vi "大富翁.vi"() -> ()   [LabVIEW 2014] (continued)
      n525 = property on="30房1" class="Bool (strict)"("Visible"=w18) -> ()  [unwired: 2 in, 2 out]
      n526 = property on="30房2" class="Bool (strict)"("Visible"=w18) -> ()  [unwired: 2 in, 2 out]
      n527 = property on="30房3" class="Bool (strict)"("Visible"=w18) -> ()  [unwired: 2 in, 2 out]
      n528 = property on="30房4" class="Bool (strict)"("Visible"=w18) -> ()  [unwired: 2 in, 2 out]
      n529 = property on="30旅1" class="Bool (strict)"("Visible"=w18) -> ()  [unwired: 2 in, 2 out]
      n530 = property on="30旅2" class="Bool (strict)"("Visible"=w18) -> ()  [unwired: 2 in, 2 out]
      n531 = property on="30旅3" class="Bool (strict)"("Visible"=w18) -> ()  [unwired: 2 in, 2 out]
      n532 = property on="30旅4" class="Bool (strict)"("Visible"=w18) -> ()  [unwired: 2 in, 2 out]
      n533 = property on="31房1" class="Bool (strict)"("Visible"=w18) -> ()  [unwired: 2 in, 2 out]
      n534 = property on="31房2" class="Bool (strict)"("Visible"=w18) -> ()  [unwired: 2 in, 2 out]
      n535 = property on="31房3" class="Bool (strict)"("Visible"=w18) -> ()  [unwired: 2 in, 2 out]
      n536 = property on="31房4" class="Bool (strict)"("Visible"=w18) -> ()  [unwired: 2 in, 2 out]
      n537 = property on="31旅1" class="Bool (strict)"("Visible"=w18) -> ()  [unwired: 2 in, 2 out]
      n538 = property on="31旅2" class="Bool (strict)"("Visible"=w18) -> ()  [unwired: 2 in, 2 out]
      n539 = property on="31旅3" class="Bool (strict)"("Visible"=w18) -> ()  [unwired: 2 in, 2 out]
      n540 = property on="31旅4" class="Bool (strict)"("Visible"=w18) -> ()  [unwired: 2 in, 2 out]
      n541 = property on="33房1" class="Bool (strict)"("Visible"=w17) -> ()  [unwired: 2 in, 2 out]
      n542 = property on="33房2" class="Bool (strict)"("Visible"=w17) -> ()  [unwired: 2 in, 2 out]
      n543 = property on="33房3" class="Bool (strict)"("Visible"=w17) -> ()  [unwired: 2 in, 2 out]
      n544 = property on="33房4" class="Bool (strict)"("Visible"=w17) -> ()  [unwired: 2 in, 2 out]
      n545 = property on="33旅1" class="Bool (strict)"("Visible"=w17) -> ()  [unwired: 2 in, 2 out]
      n546 = property on="33旅2" class="Bool (strict)"("Visible"=w17) -> ()  [unwired: 2 in, 2 out]
      n547 = property on="33旅3" class="Bool (strict)"("Visible"=w17) -> ()  [unwired: 2 in, 2 out]
      n548 = property on="33旅4" class="Bool (strict)"("Visible"=w17) -> ()  [unwired: 2 in, 2 out]
      n549 = property on="34房1" class="Bool (strict)"("Visible"=w17) -> ()  [unwired: 2 in, 2 out]
      n550 = property on="34房2" class="Bool (strict)"("Visible"=w17) -> ()  [unwired: 2 in, 2 out]
      n551 = property on="34房3" class="Bool (strict)"("Visible"=w17) -> ()  [unwired: 2 in, 2 out]
      n552 = property on="34房4" class="Bool (strict)"("Visible"=w17) -> ()  [unwired: 2 in, 2 out]
      n553 = property on="34旅1" class="Bool (strict)"("Visible"=w17) -> ()  [unwired: 2 in, 2 out]
      n554 = property on="34旅2" class="Bool (strict)"("Visible"=w17) -> ()  [unwired: 2 in, 2 out]
      n555 = property on="34旅3" class="Bool (strict)"("Visible"=w17) -> ()  [unwired: 2 in, 2 out]
      n556 = property on="34旅4" class="Bool (strict)"("Visible"=w17) -> ()  [unwired: 2 in, 2 out]
      n557 = property on="36房1" class="Bool (strict)"("Visible"=w17) -> ()  [unwired: 2 in, 2 out]
      n558 = property on="36房2" class="Bool (strict)"("Visible"=w17) -> ()  [unwired: 2 in, 2 out]
      n559 = property on="36房3" class="Bool (strict)"("Visible"=w17) -> ()  [unwired: 2 in, 2 out]
      n560 = property on="36房4" class="Bool (strict)"("Visible"=w17) -> ()  [unwired: 2 in, 2 out]
      n561 = property on="36旅1" class="Bool (strict)"("Visible"=w17) -> ()  [unwired: 2 in, 2 out]
      n562 = property on="36旅2" class="Bool (strict)"("Visible"=w17) -> ()  [unwired: 2 in, 2 out]
      n563 = property on="36旅3" class="Bool (strict)"("Visible"=w17) -> ()  [unwired: 2 in, 2 out]
      n564 = property on="36旅4" class="Bool (strict)"("Visible"=w17) -> ()  [unwired: 2 in, 2 out]
      n565 = property on="37房1" class="Bool (strict)"("Visible"=w17) -> ()  [unwired: 2 in, 2 out]
      n566 = property on="37房2" class="Bool (strict)"("Visible"=w17) -> ()  [unwired: 2 in, 2 out]
      n567 = property on="37房3" class="Bool (strict)"("Visible"=w17) -> ()  [unwired: 2 in, 2 out]
      n568 = property on="37房4" class="Bool (strict)"("Visible"=w17) -> ()  [unwired: 2 in, 2 out]
      n569 = property on="37旅1" class="Bool (strict)"("Visible"=w17) -> ()  [unwired: 2 in, 2 out]
      n570 = property on="37旅2" class="Bool (strict)"("Visible"=w17) -> ()  [unwired: 2 in, 2 out]
      n571 = property on="37旅3" class="Bool (strict)"("Visible"=w17) -> ()  [unwired: 2 in, 2 out]
      n572 = property on="37旅4" class="Bool (strict)"("Visible"=w17) -> ()  [unwired: 2 in, 2 out]
      n573 = property on="擲骰子 2" class="Bool (strict)"("Visible"=w15) -> ()  [unwired: 2 in, 2 out]
      n574 = property on="擲骰子 3" class="Bool (strict)"("Visible"=w15) -> ()  [unwired: 2 in, 2 out]
      n575 = property on="擲骰子 4" class="Bool (strict)"("Visible"=w15) -> ()  [unwired: 2 in, 2 out]
      n576 = property on="入獄 1" class="Bool (strict)"("Visible"=w15) -> ()  [unwired: 2 in, 2 out]
      n577 = property on="入獄 2" class="Bool (strict)"("Visible"=w15) -> ()  [unwired: 2 in, 2 out]
      n578 = property on="入獄 3" class="Bool (strict)"("Visible"=w15) -> ()  [unwired: 2 in, 2 out]
      n579 = property on="入獄 4" class="Bool (strict)"("Visible"=w15) -> ()  [unwired: 2 in, 2 out]
      n580 = property on="位置 1" class="DigNum (strict)"("Visible"=w15) -> ()  [unwired: 2 in, 2 out]
      n581 = property on="剩幾天 1" class="DigNum (strict)"("Visible"=w15) -> ()  [unwired: 2 in, 2 out]
      n582 = property on="位置 2" class="DigNum (strict)"("Visible"=w15) -> ()  [unwired: 2 in, 2 out]
      n583 = property on="剩幾天 2" class="DigNum (strict)"("Visible"=w15) -> ()  [unwired: 2 in, 2 out]
      n584 = property on="位置 3" class="DigNum (strict)"("Visible"=w15) -> ()  [unwired: 2 in, 2 out]
      n585 = property on="剩幾天 3" class="DigNum (strict)"("Visible"=w15) -> ()  [unwired: 2 in, 2 out]
      n586 = property on="位置 4" class="DigNum (strict)"("Visible"=w15) -> ()  [unwired: 2 in, 2 out]
      n587 = property on="剩幾天 4" class="DigNum (strict)"("Visible"=w15) -> ()  [unwired: 2 in, 2 out]
      n588 = local write "入獄 4"(w14) -> ()
      n589 = local write "入獄 3"(w14) -> ()
      n590 = local write "入獄 2"(w14) -> ()
      n591 = local write "入獄 1"(w14) -> ()
      n592 = local write "擲骰子 4"(w12) -> ()
      n593 = local write "擲骰子 3"(w12) -> ()
      n594 = local write "擲骰子 2"(w12) -> ()
      n595 = local write "擲骰子 1"(w12) -> ()
      n596 = local write "離開遊戲"(w12) -> ()
      n597 = property on="擲骰子 1" class="Bool (strict)"("DisabledEnum"=T1."Enabled" ("Disabled")) -> ()  [unwired: 2 in, 2 out]
      n598 = property on="按鈕?" class="DigNum (strict)"("Visible"=w9) -> ()  [unwired: 2 in, 2 out]
      n599 = property on="換誰?" class="DigNum (strict)"("Visible"=w9) -> ()  [unwired: 2 in, 2 out]
      n600 = property on="遊戲人數" class="DigNum (strict)"("Visible"=w9) -> ()  [unwired: 2 in, 2 out]
      n601 = local write "離開遊戲"(w9) -> ()
      n602 = property on="擲骰子 1" class="Bool (strict)"("Visible"=TRUE) -> ()  [unwired: 2 in, 2 out]
    }
    frame #1 {
      n603 = call "人數.vi"() -> ("三人 3"=w32:bool, "4"=w33:bool, "3"=w34:bool, "2"=w35:bool)  [unwired: 4 in]
      n604 = case shown="True" w32 {
        frame False {
        }
        frame True {
          w36 = u32 0 ("8機會")
          n605 = local write "5命運"(w36) -> ()
          n606 = local write "8機會"(w36) -> ()
          n607 = local write "16命運"(w36) -> ()
          n608 = local write "24機會"(w36) -> ()
          n609 = local write "28命運"(w36) -> ()
          n610 = local write "35機會"(w36) -> ()
          n611 = local write "背景"(w36) -> ()
        }
      }
      n612 = local write "白色恐怖?"(w32) -> ()
      n613 = case shown="True" w35 {
        frame False {
        }
        frame True {
          w43 = TRUE
          w44 = FALSE
          n614 = property on="玩家三財產" class="DigNum (strict)"("Visible"=w44) -> ()  [unwired: 2 in, 2 out]
          n615 = property on="P3 棋子" class="Bool (strict)"("Visible"=w44) -> ()  [unwired: 2 in, 2 out]
          n616 = property on="P3指示" class="Bool (strict)"("Visible"=w44) -> ()  [unwired: 2 in, 2 out]
          n617 = property on="玩家四財產" class="DigNum (strict)"("Visible"=w44) -> ()  [unwired: 2 in, 2 out]
          n618 = property on="P4 棋子" class="Bool (strict)"("Visible"=w44) -> ()  [unwired: 2 in, 2 out]
          n619 = property on="P4指示" class="Bool (strict)"("Visible"=w44) -> ()  [unwired: 2 in, 2 out]
          n620 = property on="玩家一財產" class="DigNum (strict)"("Visible"=w43) -> ()  [unwired: 2 in, 2 out]
          n621 = property on="P1 棋子" class="Bool (strict)"("Visible"=w43) -> ()  [unwired: 2 in, 2 out]
          n622 = property on="P1指示" class="Bool (strict)"("Visible"=w43) -> ()  [unwired: 2 in, 2 out]
          n623 = property on="玩家二財產" class="DigNum (strict)"("Visible"=w43) -> ()  [unwired: 2 in, 2 out]
          n624 = property on="P2 棋子" class="Bool (strict)"("Visible"=w43) -> ()  [unwired: 2 in, 2 out]
          n625 = property on="P2指示" class="Bool (strict)"("Visible"=w43) -> ()  [unwired: 2 in, 2 out]
          n626 = local write "遊戲人數"(2.0 ("遊戲人數")) -> ()
        }
      }
      n627 = case shown="True" w34 {
        frame False {
        }
        frame True {
          w40 = TRUE
          w41 = FALSE
          n628 = property on="玩家四財產" class="DigNum (strict)"("Visible"=w41) -> ()  [unwired: 2 in, 2 out]
          n629 = property on="P4 棋子" class="Bool (strict)"("Visible"=w41) -> ()  [unwired: 2 in, 2 out]
          n630 = property on="P4指示" class="Bool (strict)"("Visible"=w41) -> ()  [unwired: 2 in, 2 out]
          n631 = property on="玩家三財產" class="DigNum (strict)"("Visible"=w40) -> ()  [unwired: 2 in, 2 out]
          n632 = property on="P3 棋子" class="Bool (strict)"("Visible"=w40) -> ()  [unwired: 2 in, 2 out]
          n633 = property on="P3指示" class="Bool (strict)"("Visible"=w40) -> ()  [unwired: 2 in, 2 out]
          n634 = local write "遊戲人數"(3.0 ("遊戲人數")) -> ()
        }
      }
      n635 = case shown="True" w33 {
        frame False {
        }
        frame True {
          w37 = TRUE
          w38 = TRUE
          n636 = property on="玩家三財產" class="DigNum (strict)"("Visible"=w38) -> ()  [unwired: 2 in, 2 out]
          n637 = property on="P3 棋子" class="Bool (strict)"("Visible"=w38) -> ()  [unwired: 2 in, 2 out]
          n638 = property on="P3指示" class="Bool (strict)"("Visible"=w38) -> ()  [unwired: 2 in, 2 out]
          n639 = property on="玩家四財產" class="DigNum (strict)"("Visible"=w37) -> ()  [unwired: 2 in, 2 out]
          n640 = property on="P4 棋子" class="Bool (strict)"("Visible"=w37) -> ()  [unwired: 2 in, 2 out]
          n641 = property on="P4指示" class="Bool (strict)"("Visible"=w37) -> ()  [unwired: 2 in, 2 out]
          n642 = local write "遊戲人數"(4.0 ("遊戲人數")) -> ()
        }
      }
    }
    frame #2 {
      # "等按鈕"
      n643 = while {
        shift-right: [w48] -> _
        shift-left: -100 -> [w49]
        stop <- w47 stop-if-true
        # "state machine"
        n644 = case shown="-100, Default" w49 {
          selector: w49 -> [_ _ _ _ _ _ _ _ _ _ _ _ _ _ _ _ _ _ _ _ _ _ _ _ _ _ _ _ _ _ w207 w309 w410 w511 _ w956 w1057 _ w1503 w1604 w1705 w1806 _ w1909 w2009 w2110 w2212 _ w2315 w2416 w2517 w2618 w2719 w2820 w2921 w3022 w3122 w3224 _ w3348 w3449 w3550 w3651 _ _ _ _ _]
          tunnel: [w51 -100.0 ("按鈕?") -100.0 ("按鈕?") -100.0 ("按鈕?") -100.0 ("按鈕?") -100.0 ("按鈕?") -100.0 ("按鈕?") -100.0 ("按鈕?") -100.0 ("按鈕?") -100.0 ("按鈕?") -100.0 ("按鈕?") -100.0 ("按鈕?") -100.0 ("按鈕?") -100.0 ("按鈕?") -100.0 ("按鈕?") -100.0 ("按鈕?") -100.0 ("按鈕?") -100.0 ("按鈕?") -100.0 ("按鈕?") -100.0 ("按鈕?") -100.0 ("按鈕?") -100.0 ("按鈕?") -100.0 ("按鈕?") -100.0 ("按鈕?") -100.0 ("按鈕?") -100.0 ("按鈕?") -100.0 ("按鈕?") -100.0 ("按鈕?") -100.0 ("按鈕?") 42.0 ("位置 4") 42.0 ("位置 4") 42.0 ("位置 4") 42.0 ("位置 4") 42.0 ("位置 4") 42.0 ("位置 4") 42.0 ("位置 4") 42.0 ("位置 4") 42.0 ("位置 4") 42.0 ("位置 4") 42.0 ("位置 4") 42.0 ("位置 4") 42.0 ("位置 4") 42.0 ("位置 4") 42.0 ("位置 4") 42.0 ("位置 4") 42.0 ("位置 4") 42.0 ("位置 4") 42.0 ("位置 4") 42.0 ("位置 4") 42.0 ("位置 4") 42.0 ("位置 4") 42.0 ("位置 4") 42.0 ("位置 4") 42.0 ("位置 4") 42.0 ("位置 4") 42.0 ("位置 4") 42.0 ("位置 4") 42.0 ("位置 4") 42.0 ("位置 4") 42.0 ("位置 4") 42.0 ("位置 4") 42.0 ("位置 4") 42.0 ("位置 4") w3751 w3826 w3901 w3976 w4051] -> w48
          tunnel: [w50 w124 w126 w128 w130 FALSE ("苗栗縣") FALSE ("苗栗縣") FALSE ("苗栗縣") FALSE ("苗栗縣") FALSE ("苗栗縣") FALSE ("苗栗縣") FALSE ("苗栗縣") FALSE ("苗栗縣") FALSE ("苗栗縣") FALSE ("苗栗縣") FALSE ("苗栗縣") FALSE ("苗栗縣") FALSE ("苗栗縣") FALSE ("苗栗縣") FALSE ("苗栗縣") FALSE ("苗栗縣") FALSE ("苗栗縣") FALSE ("苗栗縣") FALSE ("苗栗縣") FALSE ("苗栗縣") FALSE ("苗栗縣") FALSE ("苗栗縣") FALSE ("苗栗縣") FALSE ("苗栗縣") FALSE ("苗栗縣") w206 w308 w409 w510 w610 w955 w1056 w1156 w1502 w1603 w1704 w1805 FALSE ("苗栗縣") w1908 w2010 w2111 w2211 FALSE ("苗栗縣") w2314 w2415 w2516 w2617 w2718 w2819 w2920 w3021 w3123 w3223 FALSE ("苗栗縣") w3347 w3448 w3549 w3650 FALSE ("苗栗縣") FALSE ("苗栗縣") FALSE ("苗栗縣") FALSE ("苗栗縣") FALSE ("苗栗縣")] -> w47
          frame -100, Default {
            n645 = stacked-sequence {
              tunnel: [_ w123] -> w51
              tunnel: [w52 _] -> w50
              frame #0 {
                n646 = while {
                  tunnel: [w54] -> w52
                  stop <- w84 stop-if-true
                  # "按哪個按鈕"
                  n647 = local read "中壢市"() -> (w82:bool)
                  n648 = local read "新竹市"() -> (w81:bool)
                  n649 = local read "新竹縣"() -> (w80:bool)
                  n650 = local read "苗栗縣"() -> (w79:bool)
                  n651 = local read "台中市"() -> (w78:bool)
                  n652 = local read "南投縣"() -> (w77:bool)
                  n653 = local read "彰化縣"() -> (w76:bool)
                  n654 = local read "雲林縣"() -> (w75:bool)
                  n655 = local read "嘉義市"() -> (w74:bool)
                  n656 = local read "澎湖縣"() -> (w73:bool)
                  n657 = local read "嘉義縣"() -> (w72:bool)
                  n658 = local read "阿里山"() -> (w71:bool)
                  n659 = local read "台南市"() -> (w70:bool)
                  n660 = local read "高雄市"() -> (w69:bool)
                  n661 = local read "屏東縣"() -> (w68:bool)
                  n662 = local read "小琉球"() -> (w66:bool)
                  n663 = local read "台東縣"() -> (w61:bool)
                  n664 = local read "花蓮縣"() -> (w60:bool)
                  n665 = local read "宜蘭縣"() -> (w59:bool)
                  n666 = local read "基隆市"() -> (w58:bool)
                  n667 = local read "台北市"() -> (w57:bool)
                  n668 = local read "新北市"() -> (w56:bool)
                  n669 = local read "桃園市"() -> (w55:bool)
                  n670 = local read "金門"() -> (w64:bool)
                  n671 = local read "擲骰子 4"() -> (w88:bool)
                  n672 = local read "擲骰子 3"() -> (w87:bool)
                  n673 = local read "擲骰子 2"() -> (w86:bool)
                  n674 = local read "擲骰子 1"() -> (w85:bool)
                  n675 = local read "¾Á¤B"() -> (w67:bool)
                  n676 = local read "馬祖"() -> (w65:bool)
                  n677 = local read "蘭嶼"() -> (w63:bool)
                  n678 = local read "綠島"() -> (w62:bool)
                  n679 = case shown="True" w73 {
                    frame False {
                    }
                    frame True {
                      n680 = local write "按鈕?"(-25.0 ("按鈕?")) -> ()
                    }
                  }
                  n681 = case shown="True" w64 {
                    frame False {
                    }
                    frame True {
                      n682 = local write "按鈕?"(-12.0 ("按鈕?")) -> ()
                    }
                  }
                  n683 = case shown="False" w82 {
                    frame False {
                    }
                    frame True {
                      n684 = local write "按鈕?"(-37.0 ("按鈕?")) -> ()
                    }
                  }
                  n685 = Compound Arithmetic op=OR(w88, w87, w86, w85) -> (w83:bool)
                  n686 = local read "換誰?"() -> (w53:dbl)
                  n687 = case shown="False" w81 {
                    frame False {
                    }
                    frame True {
                      n688 = local write "按鈕?"(-36.0 ("按鈕?")) -> ()
                    }
                  }
                  n689 = case shown="True" w72 {
                    frame False {
                    }
                    frame True {
                      n690 = local write "按鈕?"(-23.0 ("按鈕?")) -> ()
                    }
                  }
                  n691 = case shown="True" w63 {
                    frame False {
                    }
                    frame True {
                      n692 = local write "按鈕?"(-11.0 ("按鈕?")) -> ()
                    }
                  }
                  n693 = case shown="True" w83 {
                    tunnel: w53 -> [_ w117]
                    frame False {
                    }
                    frame True {
                      n694 = case shown="2" w117 {
                        tunnel: [38 39 40 41] -> w118
                        frame 1, Default {
                        }
                        frame 2 {
                        }
                        frame 3 {
                        }
                        frame 4 {
                        }
                      }
                      n695 = local write "按鈕?"(w118) -> ()
                    }
                  }
                  n696 = case shown="True" w80 {
                    frame False {
                    }
                    frame True {
                      n697 = local write "按鈕?"(-34.0 ("按鈕?")) -> ()
                    }
                  }
                  n698 = case shown="True" w71 {
                    frame False {
                    }
                    frame True {
                      n699 = local write "按鈕?"(-22.0 ("按鈕?")) -> ()
                    }
                  }
                  n700 = case shown="True" w62 {
                    frame False {
                    }
                    frame True {
                      n701 = local write "按鈕?"(-10.0 ("按鈕?")) -> ()
                    }
                  }
                  n702 = case shown="True" w79 {
                    frame False {
                    }
                    frame True {
                      n703 = local write "按鈕?"(-33.0 ("按鈕?")) -> ()
                    }
                  }
                  n704 = case shown="True" w70 {
                    frame False {
                    }
                    frame True {
                      n705 = local write "按鈕?"(-21.0 ("按鈕?")) -> ()
                    }
                  }
                  n706 = case shown="True" w61 {
                    frame False {
                    }
                    frame True {
                      n707 = local write "按鈕?"(-9.0 ("按鈕?")) -> ()
                    }
                  }
                  n708 = case shown="True" w78 {
                    frame False {
                    }
                    frame True {
                      n709 = local write "按鈕?"(-31.0 ("按鈕?")) -> ()
                    }
                  }
                  n710 = case shown="True" w69 {
                    frame False {
                    }
                    frame True {
                      n711 = local write "按鈕?"(-20.0 ("按鈕?")) -> ()
                    }
                  }
                  n712 = case shown="True" w60 {
                    frame False {
                    }
                    frame True {
                      n713 = local write "按鈕?"(-7.0 ("按鈕?")) -> ()
                    }
                  }
                  n714 = case shown="True" w77 {
                    frame False {
                    }
                    frame True {
                      n715 = local write "按鈕?"(-30.0 ("按鈕?")) -> ()
                    }
                  }
                  n716 = case shown="True" w68 {
                    frame False {
                    }
                    frame True {
                      n717 = local write "按鈕?"(-18.0 ("按鈕?")) -> ()
                    }
                  }
                  n718 = case shown="True" w59 {
                    frame False {
                    }
                    frame True {
                      n719 = local write "按鈕?"(-6.0 ("按鈕?")) -> ()
                    }
                  }
                  n720 = case shown="True" w76 {
                    frame False {
                    }
                    frame True {
                      n721 = local write "按鈕?"(-29.0 ("按鈕?")) -> ()
                    }
                  }
                  n722 = case shown="True" w67 {
                    frame False {
                    }
                    frame True {
                      n723 = local write "按鈕?"(-17.0 ("按鈕?")) -> ()
                    }
                  }
                  n724 = case shown="True" w58 {
                    frame False {
                    }
                    frame True {
                      n725 = local write "按鈕?"(-4.0 ("按鈕?")) -> ()
                    }
                  }
                  n726 = case shown="True" w75 {
                    frame False {
                    }
                    frame True {
                      n727 = local write "按鈕?"(-27.0 ("按鈕?")) -> ()
                    }
                  }
                  n728 = case shown="True" w66 {
                    frame False {
                    }
                    frame True {
                      n729 = local write "按鈕?"(-15.0 ("按鈕?")) -> ()
                    }
                  }
                  n730 = case shown="True" w57 {
                    frame False {
                    }
                    frame True {
                      n731 = local write "按鈕?"(-3.0 ("按鈕?")) -> ()
                    }
                  }
                  n732 = case shown="True" w74 {
                    frame False {
                    }
                    frame True {
                      n733 = local write "按鈕?"(-26.0 ("按鈕?")) -> ()
                    }
                  }
                  n734 = case shown="True" w65 {
                    frame False {
                    }
                    frame True {
                      n735 = local write "按鈕?"(-14.0 ("按鈕?")) -> ()
                    }
                  }
                  n736 = case shown="True" w56 {
                    frame False {
                    }
                    frame True {
                      n737 = local write "按鈕?"(-2.0 ("按鈕?")) -> ()
                    }
                  }
                  n738 = case shown="True" w55 {
                    frame False {
                    }
                    frame True {
                      n739 = local write "按鈕?"(-1.0 ("按鈕?")) -> ()
                    }
                  }
                  n740 = local read "離開遊戲"() -> (w54:bool)
                  n741 = Compound Arithmetic op=OR(w82, w81, w80, w79, w78, w77, w76, w75, w74, w73, w72, w71, w70, w69, w68, w67, w66, w65, w64, w63, w62, w61, w60, w59, w58, w57, w56, w55, w83, w54) -> (w84:bool)
                }
              }
              frame #1 {
                n742 = local read "按鈕?"() -> (w123:dbl)
              }
            }
          }
          frame -37 {
            w124 = FALSE ("中壢市")
            n743 = call "37查看中壢市.vi"() -> ()  [unwired: 12 in]
            n744 = local write "中壢市"(w124) -> ()
          }
          frame -36 {
            w126 = FALSE ("新竹市")
            n745 = call "36查看新竹市.vi"() -> ()  [unwired: 12 in]
            n746 = local write "新竹市"(w126) -> ()
          }
          frame -34 {
            w128 = FALSE ("新竹縣")
            n747 = call "34查看新竹縣.vi"() -> ()  [unwired: 12 in]
            n748 = local write "新竹縣"(w128) -> ()
          }
          frame -33 {
            w130 = FALSE ("苗栗縣")
            n749 = call "33查看苗栗縣.vi"() -> ()  [unwired: 12 in]
            n750 = local write "苗栗縣"(w130) -> ()
          }
          frame -31 {
            n751 = call "31查看台中市.vi"() -> ()  [unwired: 12 in]
            n752 = local write "台中市"(FALSE ("台中市")) -> ()
          }
          frame -30 {
            n753 = call "30查看南投縣.vi"() -> ()  [unwired: 12 in]
            n754 = local write "南投縣"(FALSE ("南投縣")) -> ()
          }
          frame -29 {
            n755 = call "29查看彰化縣.vi"() -> ()  [unwired: 12 in]
            n756 = local write "彰化縣"(FALSE ("彰化縣")) -> ()
          }
          frame -27 {
            n757 = call "27查看雲林縣.vi"() -> ()  [unwired: 12 in]
            n758 = local write "雲林縣"(FALSE ("雲林縣")) -> ()
          }
          frame -26 {
            n759 = call "26查看嘉義市.vi"() -> ()  [unwired: 12 in]
            n760 = local write "嘉義市"(FALSE ("嘉義市")) -> ()
          }
          frame -25 {
            n761 = call "25查看澎湖縣.vi"() -> ()  [unwired: 12 in]
            n762 = local write "澎湖縣"(FALSE ("澎湖縣")) -> ()
          }
          frame -23 {
            n763 = call "23查看嘉義縣.vi"() -> ()  [unwired: 12 in]
            n764 = local write "嘉義縣"(FALSE ("嘉義縣")) -> ()
          }
          frame -22 {
            n765 = call "22查看阿里山.vi"() -> ()  [unwired: 12 in]
            n766 = local write "阿里山"(FALSE ("阿里山")) -> ()
          }
          frame -21 {
            n767 = call "21查看台南市.vi"() -> ()  [unwired: 12 in]
            n768 = local write "台南市"(FALSE ("台南市")) -> ()
          }
          frame -20 {
            n769 = call "20查看高雄市.vi"() -> ()  [unwired: 12 in]
            n770 = local write "高雄市"(FALSE ("高雄市")) -> ()
          }
          frame -18 {
            n771 = call "18查看屏東縣.vi"() -> ()  [unwired: 12 in]
            n772 = local write "屏東縣"(FALSE ("屏東縣")) -> ()
          }
          frame -17 {
            n773 = call "17查看墾丁.vi"() -> ()  [unwired: 12 in]
            n774 = local write "¾Á¤B"(FALSE ("¾Á¤B")) -> ()
          }
          frame -15 {
            n775 = call "15查看小琉球.vi"() -> ()  [unwired: 12 in]
            n776 = local write "小琉球"(FALSE ("小琉球")) -> ()
          }
          frame -14 {
            n777 = call "14查看馬祖.vi"() -> ()  [unwired: 12 in]
            n778 = local write "馬祖"(FALSE ("馬祖")) -> ()
          }
          frame -12 {
            n779 = call "12查看金門.vi"() -> ()  [unwired: 12 in]
            n780 = local write "金門"(FALSE ("金門縣")) -> ()
          }
          frame -11 {
            n781 = call "11查看蘭嶼.vi"() -> ()  [unwired: 12 in]
            n782 = local write "蘭嶼"(FALSE ("蘭嶼")) -> ()
          }
          frame -10 {
            n783 = call "10查看綠島.vi"() -> ()  [unwired: 12 in]
            n784 = local write "綠島"(FALSE ("綠島")) -> ()
          }
          frame -9 {
            n785 = call "09查看台東縣.vi"() -> ()  [unwired: 12 in]
            n786 = local write "台東縣"(FALSE ("台東縣")) -> ()
          }
          frame -7 {
            n787 = call "07查看花蓮縣.vi"() -> ()  [unwired: 12 in]
            n788 = local write "花蓮縣"(FALSE ("花蓮縣")) -> ()
          }
          frame -6 {
            n789 = call "06查看宜蘭縣.vi"() -> ()  [unwired: 12 in]
            n790 = local write "宜蘭縣"(FALSE ("宜蘭縣")) -> ()
          }
          frame -4 {
            n791 = call "04查看基隆市.vi"() -> ()  [unwired: 12 in]
            n792 = local write "基隆市"(FALSE ("基隆市")) -> ()
          }
          frame -3 {
            n793 = call "03查看台北市.vi"() -> ()  [unwired: 12 in]
            n794 = local write "台北市"(FALSE ("台北市")) -> ()
          }
          frame -2 {
            n795 = call "02查看新北市.vi"() -> ()  [unwired: 12 in]
            n796 = local write "新北市"(FALSE ("新北市")) -> ()
          }
          frame -1 {
            n797 = call "01查看桃園市.vi"() -> ()  [unwired: 12 in]
            n798 = local write "桃園市"(FALSE ("桃園市")) -> ()
          }
          frame 0 {
            n799 = call "0起點.vi"() -> ()  [unwired: 4 in]
          }
          frame 1 {
            n800 = local read "桃園市所有"() -> (w211:u32)
            n801 = Equal?(x=w211, y=u32 16777215) -> (x = y?=w209:bool)
            n802 = case shown="False" w209 {
              tunnel: w207 -> [w231 w270]
              tunnel: [w212 FALSE] -> w206
              frame False {
                # "有主地"
                n803 = local read "換誰?"() -> (w215:dbl)
                n804 = local read "桃園市所有"() -> (w236:u32)
                n805 = call "數字轉顏色.vi"("數字"=w215) -> ("顏色數字"=w235:dbl)  [unwired: 2 in]
                n806 = case shown="4" w215 {
                  tunnel: [w265 w266 w267 w268] -> w230
                  frame 1, Default {
                    n807 = local read "玩家一財產"() -> (w265:dbl)
                  }
                  frame 2 {
                    n808 = local read "玩家二財產"() -> (w266:dbl)
                  }
                  frame 3 {
                    n809 = local read "玩家三財產"() -> (w267:dbl)
                  }
                  frame 4 {
                    n810 = local read "玩家四財產"() -> (w268:dbl)
                  }
                }
                n811 = Equal?(x=w236, y=w235) -> (x = y?=w234:bool)
                n812 = local read "1房1"() -> (w226:bool)
                n813 = local read "1房2"() -> (w225:bool)
                n814 = local read "1房3"() -> (w224:bool)
                n815 = local read "1房4"() -> (w223:bool)
                n816 = local read "1旅1"() -> (w222:bool)
                n817 = local read "1旅2"() -> (w221:bool)
                n818 = local read "1旅3"() -> (w220:bool)
                n819 = local read "1旅4"() -> (w219:bool)
                n820 = local read "桃園市所有"() -> (w218:u32)
                n821 = call "房子數量.vi"("房子 1"=w226, "房子 2"=w225, "房子 3"=w224, "房子 4"=w223, "旅館 1"=w222, "旅館 2"=w221, "旅館 3"=w220, "旅館 4"=w219) -> ("房子數"=w233:dbl, "旅館數"=w232:dbl)  [unwired: 18 in]
                n822 = call "顏色轉數字.vi"("顏色數字"=w218) -> ("數字"=w213:dbl)  [unwired: 2 in]
                n823 = case shown="1, Default" w213 {
                  tunnel: [w241 w242 w243 w244] -> w217
                  frame 1, Default {
                    n824 = local read "玩家一財產"() -> (w241:dbl)
                  }
                  frame 2 {
                    n825 = local read "玩家二財產"() -> (w242:dbl)
                  }
                  frame 3 {
                    n826 = local read "玩家三財產"() -> (w243:dbl)
                  }
                  frame 4 {
                    n827 = local read "玩家四財產"() -> (w244:dbl)
                  }
                }
                n828 = call "走到地.vi"("房子數量"=w233, "自己的地?"=w234, "旅館數量"=w232, "編號"=w231, "走到人財產"=w230) -> ("走到人-?"=w229:dbl, "蓋第幾棟"=w227:dbl, "地主+?"=w216:dbl, "破產?"=w212:bool)
                n829 = Subtract(x=w230, y=w229) -> (x-y=w228:dbl)
                n830 = Add(x=w216, y=w217) -> (x+y=w214:dbl)
                n831 = case shown="1, Default" w213 {
                  tunnel: w214 -> [w237 w238 w239 w240]
                  frame 1, Default {
                    n832 = local write "玩家一財產"(w237) -> ()
                  }
                  frame 2 {
                    n833 = local write "玩家二財產"(w238) -> ()
                  }
                  frame 3 {
                    n834 = local write "玩家三財產"(w239) -> ()
                  }
                  frame 4 {
                    n835 = local write "玩家四財產"(w240) -> ()
                  }
                }
                n836 = case shown="7" w227 {
                  frame 0, Default {
                  }
                  frame 1 {
                    n837 = flat-sequence {
                      frame #0 {
                        n838 = local write "1房1"(TRUE ("1房1")) -> ()
                      }
                      frame #1 {
                        n839 = property on="1房1" class="Bool (strict)"("Visible"=TRUE) -> ()  [unwired: 2 in, 2 out]
                      }
                    }
                  }
                  frame 2 {
                    n840 = flat-sequence {
                      frame #0 {
                        n841 = local write "1房2"(TRUE ("1房2")) -> ()
                      }
                      frame #1 {
                        n842 = property on="1房2" class="Bool (strict)"("Visible"=TRUE ("1房2")) -> ()  [unwired: 2 in, 2 out]
                      }
                    }
                  }
                  frame 3 {
                    n843 = flat-sequence {
                      frame #0 {
                        n844 = local write "1房3"(TRUE) -> ()
                      }
                      frame #1 {
                        n845 = property on="1房3" class="Bool (strict)"("Visible"=TRUE) -> ()  [unwired: 2 in, 2 out]
                      }
                    }
                  }
                  frame 4 {
                    n846 = flat-sequence {
                      frame #0 {
                        n847 = local write "1房4"(TRUE) -> ()
                      }
                      frame #1 {
                        n848 = property on="1房4" class="Bool (strict)"("Visible"=TRUE) -> ()  [unwired: 2 in, 2 out]
                      }
                    }
                  }
                  frame 5 {
                    n849 = flat-sequence {
                      frame #0 {
                        n850 = local write "1旅1"(TRUE) -> ()
                      }
                      frame #1 {
                        n851 = property on="1旅1" class="Bool (strict)"("Visible"=TRUE) -> ()  [unwired: 2 in, 2 out]
                      }
                    }
                  }
                  frame 6 {
                    n852 = flat-sequence {
                      frame #0 {
                        n853 = local write "1旅2"(TRUE) -> ()
                      }
                      frame #1 {
                        n854 = property on="1旅2" class="Bool (strict)"("Visible"=TRUE) -> ()  [unwired: 2 in, 2 out]
                      }
                    }
                  }
                  frame 7 {
                    n855 = flat-sequence {
                      frame #0 {
                        n856 = local write "1旅3"(TRUE) -> ()
                      }
                      frame #1 {
                        n857 = property on="1旅3" class="Bool (strict)"("Visible"=TRUE) -> ()  [unwired: 2 in, 2 out]
                      }
                    }
                  }
                  frame 8 {
                    n858 = flat-sequence {
                      frame #0 {
                        n859 = local write "1旅4"(TRUE) -> ()
                      }
                      frame #1 {
                        n860 = property on="1旅4" class="Bool (strict)"("Visible"=TRUE) -> ()  [unwired: 2 in, 2 out]
                      }
                    }
                  }
                }
                n861 = case shown="1, Default" w215 {
                  tunnel: w228 -> [w261 w262 w263 w264]
                  frame 1, Default {
                    n862 = local write "玩家一財產"(w261) -> ()
                  }
                  frame 2 {
                    n863 = local write "玩家二財產"(w262) -> ()
                  }
                  frame 3 {
                    n864 = local write "玩家三財產"(w263) -> ()
                  }
                  frame 4 {
                    n865 = local write "玩家四財產"(w264) -> ()
                  }
                }
              }
              frame True {
                # "無主地"
                n866 = call "購買土地.vi"() -> ("確定 2"=w271:bool)  [unwired: 3 in]
                n867 = case shown="True" w271 {
                  tunnel: w270 -> [_ w275]
                  frame False {
                    # "不買"
                  }
                  frame True {
                    # "要買"
                    n868 = local read "換誰?"() -> (w276:dbl)
                    n869 = case shown="4" w276 {
                      tunnel: [w303 w304 w305 w306] -> w274
                      frame 1, Default {
                        n870 = local read "玩家一財產"() -> (w303:dbl)
                      }
                      frame 2 {
                        n871 = local read "玩家二財產"() -> (w304:dbl)
                      }
                      frame 3 {
                        n872 = local read "玩家三財產"() -> (w305:dbl)
                      }
                      frame 4 {
                        n873 = local read "玩家四財產"() -> (w306:dbl)
                      }
                    }
                    n874 = call "各種價格.vi"("Numeric"=w275) -> ("買空地"=w273:dbl)  [unwired: 4 in, 5 out]
                    n875 = Greater Or Equal?(x=w274, y=w273) -> (x >= y?=w272:bool)
                    n876 = case shown="True" w272 {
                      tunnel: w275 -> [_ w277]
                      frame False {
                        # "錢不夠"
                        n877 = call "錢不夠.vi"() -> ()  [unwired: 4 in]
                      }
                      frame True {
                        # "錢夠"
                        n878 = local read "換誰?"() -> (w278:dbl)
                        n879 = case shown="4" w278 {
                          selector: w278 -> [w282 w288 w294 w300]
                          tunnel: w277 -> [w281 w287 w293 w299]
                          frame 1, Default {
                            # "誰買了地"
                            n880 = call "各種價格.vi"("Numeric"=w281) -> ("買空地"=w280:dbl)  [unwired: 4 in, 5 out]
                            n881 = local read "玩家一財產"() -> (w284:dbl)
                            n882 = Subtract(x=w284, y=w280) -> (x-y=w283:dbl)
                            n883 = local write "玩家一財產"(w283) -> ()
                            n884 = call "數字轉顏色.vi"("數字"=w282) -> ("顏色數字"=w279:dbl)  [unwired: 2 in]
                            n885 = local write "桃園市所有"(w279) -> ()
                            n886 = local write "1桃園市"(w279) -> ()
                          }
                          frame 2 {
                            # "誰買了地"
                            n887 = call "各種價格.vi"("Numeric"=w287) -> ("買空地"=w286:dbl)  [unwired: 4 in, 5 out]
                            n888 = local read "玩家二財產"() -> (w290:dbl)
                            n889 = Subtract(x=w290, y=w286) -> (x-y=w289:dbl)
                            n890 = local write "玩家二財產"(w289) -> ()
                            n891 = call "數字轉顏色.vi"("數字"=w288) -> ("顏色數字"=w285:dbl)  [unwired: 2 in]
                            n892 = local write "桃園市所有"(w285) -> ()
                            n893 = local write "1桃園市"(w285) -> ()
                          }
                          frame 3 {
                            # "誰買了地"
                            n894 = local read "玩家三財產"() -> (w295:dbl)
                            n895 = call "各種價格.vi"("Numeric"=w293) -> ("買空地"=w292:dbl)  [unwired: 4 in, 5 out]
                            n896 = Subtract(x=w295, y=w292) -> (x-y=w296:dbl)
                            n897 = call "數字轉顏色.vi"("數字"=w294) -> ("顏色數字"=w291:dbl)  [unwired: 2 in]
                            n898 = local write "玩家三財產"(w296) -> ()
                            n899 = local write "桃園市所有"(w291) -> ()
                            n900 = local write "1桃園市"(w291) -> ()
                          }
                          frame 4 {
                            # "誰買了地"
                            n901 = call "各種價格.vi"("Numeric"=w299) -> ("買空地"=w298:dbl)  [unwired: 4 in, 5 out]
                            n902 = local read "玩家四財產"() -> (w302:dbl)
                            n903 = Subtract(x=w302, y=w298) -> (x-y=w301:dbl)
                            n904 = local write "玩家四財產"(w301) -> ()
                            n905 = call "數字轉顏色.vi"("數字"=w300) -> ("顏色數字"=w297:dbl)  [unwired: 2 in]
                            n906 = local write "1桃園市"(w297) -> ()
                            n907 = local write "桃園市所有"(w297) -> ()
                          }
                        }
                      }
                    }
                  }
                }
              }
            }
          }
          frame 2 {
            n908 = local read "新北市所有"() -> (w307:u32)
            n909 = Equal?(x=w307, y=u32 16777215) -> (x = y?=w310:bool)
            n910 = case shown="False" w310 {
              tunnel: w309 -> [w333 w371]
              tunnel: [w323 FALSE] -> w308
              frame False {
                # "有主地"
                n911 = local read "換誰?"() -> (w326:dbl)
                n912 = local read "新北市所有"() -> (w322:u32)
                n913 = call "數字轉顏色.vi"("數字"=w326) -> ("顏色數字"=w337:dbl)  [unwired: 2 in]
                n914 = case shown="4" w326 {
                  tunnel: [w366 w367 w368 w369] -> w332
                  frame 1, Default {
                    n915 = local read "玩家一財產"() -> (w366:dbl)
                  }
                  frame 2 {
                    n916 = local read "玩家二財產"() -> (w367:dbl)
                  }
                  frame 3 {
                    n917 = local read "玩家三財產"() -> (w368:dbl)
                  }
                  frame 4 {
                    n918 = local read "玩家四財產"() -> (w369:dbl)
                  }
                }
                n919 = Equal?(x=w322, y=w337) -> (x = y?=w336:bool)
                n920 = local read "新北市所有"() -> (w313:u32)
                n921 = local read "2房1"() -> (w321:bool)
                n922 = local read "2房2"() -> (w320:bool)
                n923 = local read "2房3"() -> (w319:bool)
                n924 = local read "2房4"() -> (w318:bool)
                n925 = local read "2旅1"() -> (w317:bool)
                n926 = local read "2旅2"() -> (w316:bool)
                n927 = local read "2旅3"() -> (w315:bool)
                n928 = local read "2旅4"() -> (w314:bool)
                n929 = call "房子數量.vi"("房子 1"=w321, "房子 2"=w320, "房子 3"=w319, "房子 4"=w318, "旅館 1"=w317, "旅館 2"=w316, "旅館 3"=w315, "旅館 4"=w314) -> ("房子數"=w335:dbl, "旅館數"=w334:dbl)  [unwired: 18 in]
                n930 = call "顏色轉數字.vi"("顏色數字"=w313) -> ("數字"=w324:dbl)  [unwired: 2 in]
                n931 = case shown="1, Default" w324 {
                  tunnel: [w342 w343 w344 w345] -> w328
                  frame 1, Default {
                    n932 = local read "玩家一財產"() -> (w342:dbl)
                  }
                  frame 2 {
                    n933 = local read "玩家二財產"() -> (w343:dbl)
                  }
                  frame 3 {
                    n934 = local read "玩家三財產"() -> (w344:dbl)
                  }
                  frame 4 {
                    n935 = local read "玩家四財產"() -> (w345:dbl)
                  }
                }
                n936 = call "走到地.vi"("房子數量"=w335, "自己的地?"=w336, "旅館數量"=w334, "編號"=w333, "走到人財產"=w332) -> ("走到人-?"=w331:dbl, "蓋第幾棟"=w329:dbl, "地主+?"=w327:dbl, "破產?"=w323:bool)
                n937 = Subtract(x=w332, y=w331) -> (x-y=w330:dbl)
                n938 = Add(x=w327, y=w328) -> (x+y=w325:dbl)
                n939 = case shown="1, Default" w324 {
                  tunnel: w325 -> [w338 w339 w340 w341]
                  frame 1, Default {
                    n940 = local write "玩家一財產"(w338) -> ()
                  }
                  frame 2 {
                    n941 = local write "玩家二財產"(w339) -> ()
                  }
                  frame 3 {
                    n942 = local write "玩家三財產"(w340) -> ()
                  }
                  frame 4 {
                    n943 = local write "玩家四財產"(w341) -> ()
                  }
                }
                n944 = case shown="8" w329 {
                  frame 0, Default {
                  }
                  frame 1 {
                    n945 = flat-sequence {
                      frame #0 {
                        n946 = local write "2房1"(TRUE ("1房1")) -> ()
                      }
                      frame #1 {
                        n947 = property on="2房1" class="Bool (strict)"("Visible"=TRUE) -> ()  [unwired: 2 in, 2 out]
                      }
                    }
                  }
                  frame 2 {
                    n948 = flat-sequence {
                      frame #0 {
                        n949 = local write "2房2"(TRUE ("2房2")) -> ()
                      }
                      frame #1 {
                        n950 = property on="2房2" class="Bool (strict)"("Visible"=TRUE) -> ()  [unwired: 2 in, 2 out]
                      }
                    }
                  }
                  frame 3 {
                    n951 = flat-sequence {
                      frame #0 {
                        n952 = local write "2房3"(TRUE) -> ()
                      }
                      frame #1 {
                        n953 = property on="2房3" class="Bool (strict)"("Visible"=TRUE) -> ()  [unwired: 2 in, 2 out]
                      }
                    }
                  }
                  frame 4 {
                    n954 = flat-sequence {
                      frame #0 {
                        n955 = local write "2房4"(TRUE) -> ()
                      }
                      frame #1 {
                        n956 = property on="2房4" class="Bool (strict)"("Visible"=TRUE) -> ()  [unwired: 2 in, 2 out]
                      }
                    }
                  }
                  frame 5 {
                    n957 = flat-sequence {
                      frame #0 {
                        n958 = local write "2旅1"(TRUE) -> ()
                      }
                      frame #1 {
                        n959 = property on="2旅1" class="Bool (strict)"("Visible"=TRUE) -> ()  [unwired: 2 in, 2 out]
                      }
                    }
                  }
                  frame 6 {
                    n960 = flat-sequence {
                      frame #0 {
                        n961 = local write "2旅2"(TRUE) -> ()
                      }
                      frame #1 {
                        n962 = property on="2旅2" class="Bool (strict)"("Visible"=TRUE) -> ()  [unwired: 2 in, 2 out]
                      }
                    }
                  }
                  frame 7 {
                    n963 = flat-sequence {
                      frame #0 {
                        n964 = local write "2旅3"(TRUE) -> ()
                      }
                      frame #1 {
                        n965 = property on="2旅3" class="Bool (strict)"("Visible"=TRUE) -> ()  [unwired: 2 in, 2 out]
                      }
                    }
                  }
                  frame 8 {
                    n966 = flat-sequence {
                      frame #0 {
                        n967 = local write "2旅4"(TRUE) -> ()
                      }
                      frame #1 {
                        n968 = property on="2旅4" class="Bool (strict)"("Visible"=TRUE) -> ()  [unwired: 2 in, 2 out]
                      }
                    }
                  }
                }
                n969 = case shown="1, Default" w326 {
                  tunnel: w330 -> [w362 w363 w364 w365]
                  frame 1, Default {
                    n970 = local write "玩家一財產"(w362) -> ()
                  }
                  frame 2 {
                    n971 = local write "玩家二財產"(w363) -> ()
                  }
                  frame 3 {
                    n972 = local write "玩家三財產"(w364) -> ()
                  }
                  frame 4 {
                    n973 = local write "玩家四財產"(w365) -> ()
                  }
                }
              }
              frame True {
                # "無主地"
                n974 = call "購買土地.vi"() -> ("確定 2"=w372:bool)  [unwired: 3 in]
                n975 = case shown="True" w372 {
                  tunnel: w371 -> [_ w376]
                  frame False {
                    # "不買"
                  }
                  frame True {
                    # "要買"
                    n976 = local read "換誰?"() -> (w377:dbl)
                    n977 = case shown="4" w377 {
                      tunnel: [w404 w405 w406 w407] -> w375
                      frame 1, Default {
                        n978 = local read "玩家一財產"() -> (w404:dbl)
                      }
                      frame 2 {
                        n979 = local read "玩家二財產"() -> (w405:dbl)
                      }
                      frame 3 {
                        n980 = local read "玩家三財產"() -> (w406:dbl)
                      }
                      frame 4 {
                        n981 = local read "玩家四財產"() -> (w407:dbl)
                      }
                    }
                    n982 = call "各種價格.vi"("Numeric"=w376) -> ("買空地"=w374:dbl)  [unwired: 4 in, 5 out]
                    n983 = Greater Or Equal?(x=w375, y=w374) -> (x >= y?=w373:bool)
                    n984 = case shown="True" w373 {
                      tunnel: w376 -> [_ w378]
                      frame False {
                        # "錢不夠"
                        n985 = call "錢不夠.vi"() -> ()  [unwired: 4 in]
                      }
                      frame True {
                        # "錢夠"
                        n986 = local read "換誰?"() -> (w379:dbl)
                        n987 = case shown="4" w379 {
                          selector: w379 -> [w383 w389 w395 w401]
                          tunnel: w378 -> [w382 w388 w394 w400]
                          frame 1, Default {
                            # "誰買了地"
                            n988 = call "各種價格.vi"("Numeric"=w382) -> ("買空地"=w381:dbl)  [unwired: 4 in, 5 out]
                            n989 = local read "玩家一財產"() -> (w385:dbl)
                            n990 = Subtract(x=w385, y=w381) -> (x-y=w384:dbl)
                            n991 = local write "玩家一財產"(w384) -> ()
                            n992 = call "數字轉顏色.vi"("數字"=w383) -> ("顏色數字"=w380:dbl)  [unwired: 2 in]
                            n993 = local write "2新北市"(w380) -> ()
                            n994 = local write "新北市所有"(w380) -> ()
                          }
                          frame 2 {
                            # "誰買了地"
                            n995 = call "各種價格.vi"("Numeric"=w388) -> ("買空地"=w387:dbl)  [unwired: 4 in, 5 out]
                            n996 = local read "玩家二財產"() -> (w391:dbl)
                            n997 = Subtract(x=w391, y=w387) -> (x-y=w390:dbl)
                            n998 = local write "玩家二財產"(w390) -> ()
                            n999 = call "數字轉顏色.vi"("數字"=w389) -> ("顏色數字"=w386:dbl)  [unwired: 2 in]
                            n1000 = local write "2新北市"(w386) -> ()
                            n1001 = local write "新北市所有"(w386) -> ()
                          }
                          frame 3 {
                            # "誰買了地"
                            n1002 = local read "玩家三財產"() -> (w396:dbl)
                            n1003 = call "各種價格.vi"("Numeric"=w394) -> ("買空地"=w393:dbl)  [unwired: 4 in, 5 out]
                            n1004 = Subtract(x=w396, y=w393) -> (x-y=w397:dbl)
                            n1005 = call "數字轉顏色.vi"("數字"=w395) -> ("顏色數字"=w392:dbl)  [unwired: 2 in]
                            n1006 = local write "玩家三財產"(w397) -> ()
                            n1007 = local write "2新北市"(w392) -> ()
                            n1008 = local write "新北市所有"(w392) -> ()
                          }
                          frame 4 {
                            # "誰買了地"
                            n1009 = call "各種價格.vi"("Numeric"=w400) -> ("買空地"=w399:dbl)  [unwired: 4 in, 5 out]
                            n1010 = local read "玩家四財產"() -> (w403:dbl)
                            n1011 = Subtract(x=w403, y=w399) -> (x-y=w402:dbl)
                            n1012 = local write "玩家四財產"(w402) -> ()
                            n1013 = call "數字轉顏色.vi"("數字"=w401) -> ("顏色數字"=w398:dbl)  [unwired: 2 in]
                            n1014 = local write "2新北市"(w398) -> ()
                            n1015 = local write "新北市所有"(w398) -> ()
                          }
                        }
                      }
                    }
                  }
                }
              }
            }
          }
          frame 3 {
            n1016 = local read "台北市所有"() -> (w408:u32)
            n1017 = Equal?(x=w408, y=u32 16777215) -> (x = y?=w411:bool)
            n1018 = case shown="False" w411 {
              tunnel: w410 -> [w434 w472]
              tunnel: [w424 FALSE] -> w409
              frame False {
                # "有主地"
                n1019 = local read "換誰?"() -> (w427:dbl)
                n1020 = local read "台北市所有"() -> (w423:u32)
                n1021 = call "數字轉顏色.vi"("數字"=w427) -> ("顏色數字"=w438:dbl)  [unwired: 2 in]
                n1022 = case shown="4" w427 {
                  tunnel: [w467 w468 w469 w470] -> w433
                  frame 1, Default {
                    n1023 = local read "玩家一財產"() -> (w467:dbl)
                  }
                  frame 2 {
                    n1024 = local read "玩家二財產"() -> (w468:dbl)
                  }
                  frame 3 {
                    n1025 = local read "玩家三財產"() -> (w469:dbl)
                  }
                  frame 4 {
                    n1026 = local read "玩家四財產"() -> (w470:dbl)
                  }
                }
                n1027 = Equal?(x=w423, y=w438) -> (x = y?=w437:bool)
                n1028 = local read "台北市所有"() -> (w422:u32)
                n1029 = local read "3房1"() -> (w421:bool)
                n1030 = local read "3房2"() -> (w420:bool)
                n1031 = local read "3房3"() -> (w414:bool)
                n1032 = local read "3房4"() -> (w419:bool)
                n1033 = local read "3旅1"() -> (w418:bool)
                n1034 = local read "3旅2"() -> (w417:bool)
                n1035 = local read "3旅3"() -> (w416:bool)
                n1036 = local read "3旅4"() -> (w415:bool)
                n1037 = call "房子數量.vi"("房子 1"=w421, "房子 2"=w420, "房子 3"=w414, "房子 4"=w419, "旅館 1"=w418, "旅館 2"=w417, "旅館 3"=w416, "旅館 4"=w415) -> ("房子數"=w436:dbl, "旅館數"=w435:dbl)  [unwired: 18 in]
